vi "start.vi"(8 "error in (no error)":errorcluster, 11 "PressureValve in":refnum<class "PressureValve.lvclass">) -> (0 "error out":errorcluster, 3 "PressureValve out":refnum<class "PressureValve.lvclass">)   [LabVIEW 2015, in "PressureValve.lvlib" / "PressureValve.lvclass"]
uses:
  <userlib>/Common/Devices/PressureValve/PressureValve/PressureValve.lvclass
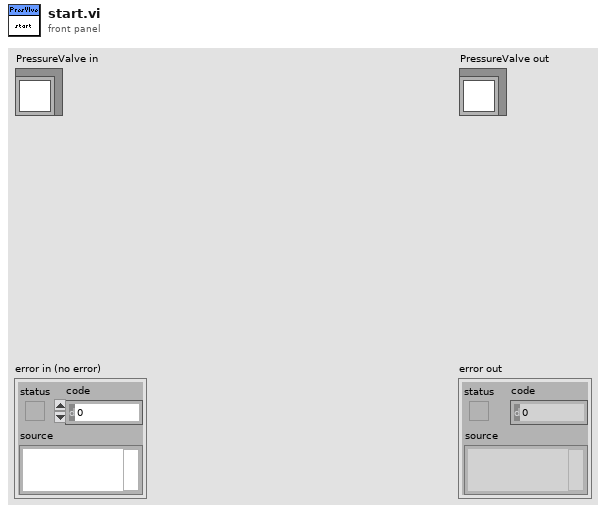
[diagram p1: front panel]
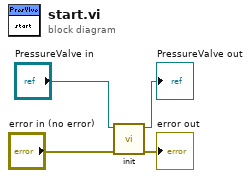
[diagram p0: block diagram]
diagram:
  n1 = call-dynamic "init.vi"("error in (no error)"="error in (no error)", "PressureValve in"="PressureValve in") -> ("error out"=→"error out":errorcluster, "PressureValve out"=→"PressureValve out":refnum<class "PressureValve.lvclass">)  [unwired: 8 in]
